vi "Terminal Attributes Descending Order.vi"(10 "Terminal Attributes":T2) -> (1 "Attributes Descending Order":T1[](array[typedef]), 2 "Terminal Descending Order":i32[](array[numeric]))   [LabVIEW 2020, in "_Rescript.lvlib"]
uses:
  _Rescript.lvlib
  Attributes.ctl
  Terminal Attributes.ctl
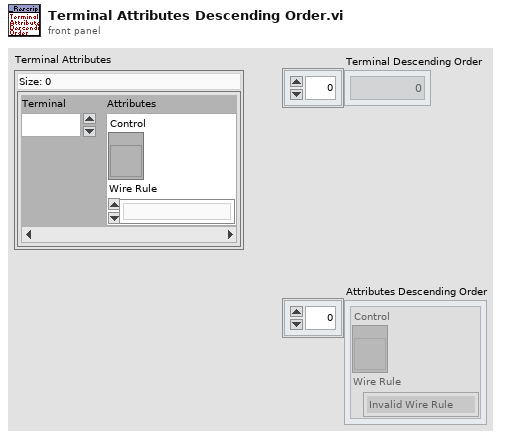
[diagram p1: front panel]
types:
  T1 = typedef "_Rescript.lvlib/Attributes.ctl" = cluster{"Control":refnum<vi>, "Wire Rule":enum16{"Invalid Wire Rule", "Required", "Recommended", "Optional", "Dynamic Dispatch"}}
  T2 = typedef "_Rescript.lvlib/Terminal Attributes.ctl" = map{i32, T1}
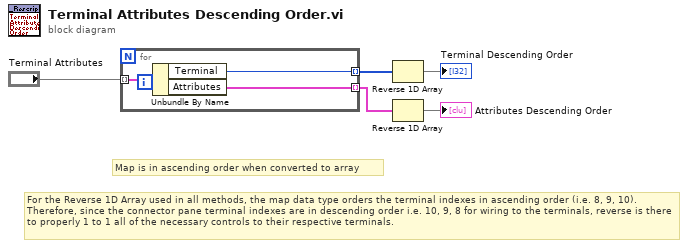
[diagram p0: block diagram]
diagram:
  # "For the Reverse 1D Array used in all methods, the map data type orders the terminal indexes in ascending order (i.e. 8, 9, 10). Therefore, since the connector pane terminal indexes are in descending order i.e. 10, 9, 8 for wiring to the terminals, reverse is there to properly 1 to 1 all of the necessary controls to their respective terminals."
  # "Map is in ascending order when converted to array"
  n1 = for {
    tunnel: "Terminal Attributes" -> [w8] mode=indexing
    tunnel: [w7] -> w4 mode=indexing
    tunnel: [w6] -> w3 mode=indexing
    n2 = Unbundle By Name(w8) -> ("Terminal"=w7:i32, "Attributes"=w6:T1)
  }
  n3 = Reverse 1D Array(array=w4) -> (reversed array=→"Terminal Descending Order":i32[])
  n4 = Reverse 1D Array(array=w3) -> (reversed array=→"Attributes Descending Order":T1[])
